vi "INIT.vi"(8 "error in (no error)":errorcluster, 11 "UV-VIS_AVANTES in":refnum<class "UV-VIS_AVANTES.lvclass">) -> (0 "error out":errorcluster, 3 "UV-VIS_AVANTES out":refnum<class "UV-VIS_AVANTES.lvclass">)   [LabVIEW 2020, in "UV-VIS_AVANTES.lvclass"]
uses:
  UV-VIS_AVANTES.lvclass
  C:/dev/TRANCON/Classes/GeneralFunctionality/GeneralFunctionality.lvclass
  C:/dev/TRANCON/Classes/Detector/Detector.lvclass
  GeneralFunctionality/GeneralFunctionality.lvclass/GeneralFunctionality.ctl
  UV-VIS_AVANTES.lvclass/UV-VIS_AVANTES.ctl
  Detector.lvclass/Detector.ctl
  dependecies/globalVarII.vi
  Config/Config.lvclass
  Detector.lvclass
  GeneralFunctionality/GeneralFunctionality.lvclass
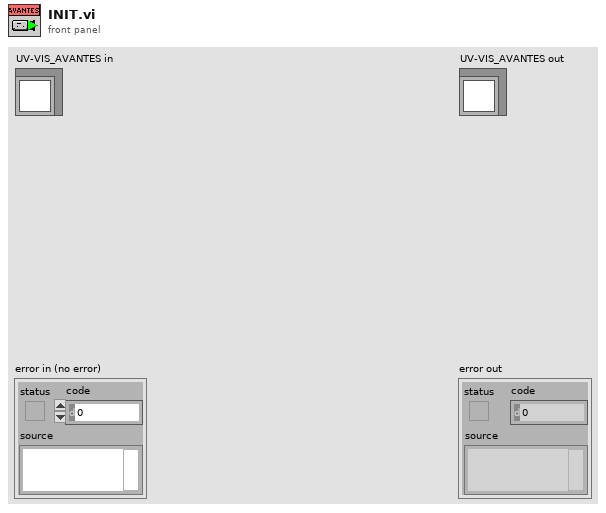
[diagram p1: front panel]
types:
  T1 = typedef "UV-VIS_AVANTES.lvclass/def_parameters.ctl" = cluster{"Len":u16, "ConfigVersion":u16, "UserFriendlyId":u8[], "DetectorType":cluster{"SensorType":u8, "NrPixels":u16, "Fit":sgl[], "NLEnable":u8, "NLCorrect":dbl[], "LowNLCounts":dbl, "HighNLCounts":dbl, "Gain":sgl[], "Reserved":sgl, "Offset":sgl[], "Extern Offset":sgl, "DefectivePixels":u16[]}, "IrradianceType":cluster{"SpectrumCalibrationType":cluster{"SmoothingType":cluster{"m_SmoothPix":u16, "SmoothModel":u8}, "CalInttime":sgl, "CalibConvers":sgl[]}, "CalibrationType":u8, "FiberDiameter":i32}, "SpectrumCalibrationType":cluster{"SmoothingType":cluster{"m_SmoothPix":u16, "SmoothModel":u8}, "CalInttime":sgl, "CalibConvers":sgl[]}, "SpectrumCorrectionType":sgl[], "StandAloneType":cluster{"StandAloneType":u8, "MeasConfigType":cluster{"StartPixel":u16, "StopPixel":u16, "IntegrationTime":sgl, "IntegrationDelay":u32, "NrAverages":u32, "DarkCorrectionType":cluster{"Enable CorDynDark":u8, "ForgetPercentage":u8}, "SmoothingType":cluster{"SmoothPix":u16, "SmoothModel":u8}, "SatDetection":u8, "TriggerType":cluster{"Trigger Mode":u8, "Trigger Source":u8, "Trigger SourceType":u8}, "ControlSettingsType":cluster{"StrobeControl":u16, "LaserDelay":u32, "LaserWidth":u32, "LaserWaveLength":sgl, "StoreToRam":u16}}, "Nmsr":i16}, "DynamicStorageType":cluster{"Nmsr":i32, "Reserved":u8[]}, "TempSensorType":sgl[], "TecControlType":cluster{"Enable":u8, "Setpoint":sgl, "Fit[NR_DAC_POL_COEF]":sgl[]}, "ProcessControlType":cluster{"AnalogLow":sgl[], "AnalogHigh":sgl[], "DigitalLow":sgl[], "DigitalHigh":sgl[]}, "EthernetSettingsType":cluster{"IpAddr":u32, "NetMask":u32, "Gateway":u32, "DhcpEnabled":u8, "TcpPort":u16, "LinkStatus":u8}, "Reserved":u8[]}
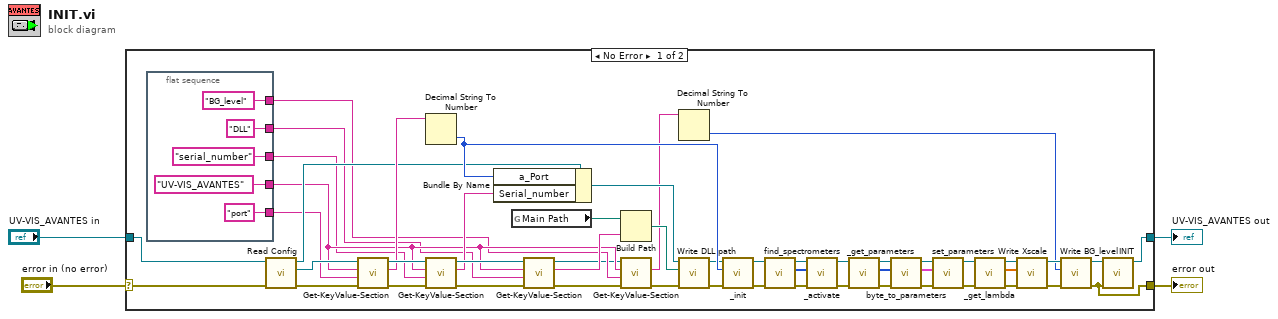
[diagram p0: block diagram]
diagram:
  n1 = case shown="No Error" "error in (no error)" {
    selector: "error in (no error)" -> [w44 w61]
    tunnel: [w32 w62] -> w3
    tunnel: "UV-VIS_AVANTES in" -> [w50 w62]
    tunnel: [w5 w61] -> w1
    frame No Error {
      n2 = flat-sequence {
        tunnel: ["UV-VIS_AVANTES" ("Section")] -> w11
        tunnel: ["serial_number" ("Key")] -> w10
        tunnel: ["BG_level" ("Key")] -> w9
        tunnel: ["port" ("Key")] -> w8
        tunnel: ["DLL" ("Key")] -> w7
        frame #0 {
        }
      }
      n3 = call "Read Config.vi"("error in (no error)"=w44, "GeneralFunctionality en entrée"=w50) -> ("error out"=w49:errorcluster, "Config.lvclass"=w51:refnum<class "Config.lvclass">, "GeneralFunctionality en sortie"=w43:refnum<class "UV-VIS_AVANTES.lvclass">)  [unwired: 7 in]
      n4 = call-dynamic "Get-KeyValue-Section.vi"("error in (no error)"=w49, "Key"=w8, "Section"=w11, "Config in"=w51) -> ("error out"=w48:errorcluster, "Value"=w46:string, "Config out"=w47:refnum<class "Config.lvclass">)  [unwired: 5 in]
      n5 = Decimal String To Number(string=w46) -> (number=w45:i32)  [unwired: 2 in, 1 out]
      n6 = call-dynamic "Get-KeyValue-Section.vi"("error in (no error)"=w48, "Key"=w10, "Section"=w11, "Config in"=w47) -> ("error out"=w28:errorcluster, "Value"=w19:string, "Config out"=w27:refnum<class "Config.lvclass">)  [unwired: 5 in]
      n7 = Bundle By Name(cluster=w43, "a_Port"=w45, "Serial_number"=w19) -> (w31:refnum<class "UV-VIS_AVANTES.lvclass">)
      n8 = global read "globalVarII.vi" "Main Path"() -> (w20:path)
      n9 = call-dynamic "Get-KeyValue-Section.vi"("error in (no error)"=w28, "Key"=w7, "Section"=w11, "Config in"=w27) -> ("error out"=w15:errorcluster, "Value"=w26:string, "Config out"=w6:refnum<class "Config.lvclass">)  [unwired: 5 in]
      n10 = Build Path(base path=w20, name or relative path=w26) -> (appended path=w25:path)
      n11 = call-dynamic "Get-KeyValue-Section.vi"("error in (no error)"=w15, "Key"=w9, "Section"=w11, "Config in"=w6) -> ("error out"=w14:errorcluster, "Value"=w13:string)  [unwired: 5 in, 1 out]
      n12 = Decimal String To Number(string=w13) -> (number=w12:i32)  [unwired: 2 in, 1 out]
      n13 = call "Write DLL path.vi"("error in (no error)"=w14, "DLL path"=w25, "Detector in"=w31) -> ("error out"=w29:errorcluster, "Detector out"=w30:refnum<class "UV-VIS_AVANTES.lvclass">)  [unwired: 7 in]
      n14 = call "_init.vi"("error in (no error)"=w29, "a_Port"=w45, "UV-VIS_AVANTES in"=w30) -> ("error out"=w53:errorcluster, "UV-VIS_AVANTES out"=w54:refnum<class "UV-VIS_AVANTES.lvclass">)  [unwired: 6 in, 1 out]
      n15 = call "find_spectrometers.vi"("error in (no error)"=w53, "UV-VIS_AVANTES in"=w54) -> ("error out"=w52:errorcluster, "List Output"=w42:u8[], "UV-VIS_AVANTES out"=w55:refnum<class "UV-VIS_AVANTES.lvclass">)  [unwired: 7 in]
      n16 = call "_activate.vi"("error in (no error)"=w52, "a_pDeviceId IN"=w42, "UV-VIS_AVANTES in"=w55) -> ("error out"=w36:errorcluster, "UV-VIS_AVANTES out"=w37:refnum<class "UV-VIS_AVANTES.lvclass">)  [unwired: 7 in]
      n17 = call "_get_parameters.vi"("error in (no error)"=w36, "UV-VIS_AVANTES in"=w37) -> ("error out"=w41:errorcluster, "DeviceParam"=w21:u8[], "UV-VIS_AVANTES out"=w38:refnum<class "UV-VIS_AVANTES.lvclass">)  [unwired: 7 in]
      n18 = call "byte_to_parameters.vi"("error in (no error)"=w41, "DeviceParam"=w21, "UV-VIS_AVANTES in"=w38) -> ("error out"=w39:errorcluster, "parameters cluster"=w24:T1, "UV-VIS_AVANTES out"=w40:refnum<class "UV-VIS_AVANTES.lvclass">)  [unwired: 6 in]
      n19 = call "set_parameters.vi"("error in (no error)"=w39, "AVS_parameters"=w24, "UV-VIS_AVANTES in"=w40) -> ("error out"=w22:errorcluster, "UV-VIS_AVANTES out"=w23:refnum<class "UV-VIS_AVANTES.lvclass">)  [unwired: 7 in]
      n20 = call "_get_lambda.vi"("error in (no error)"=w22, "UV-VIS_AVANTES in"=w23) -> ("error out"=w33:errorcluster, "a_pWaveLength"=w35:dbl[], "UV-VIS_AVANTES out"=w34:refnum<class "UV-VIS_AVANTES.lvclass">)  [unwired: 7 in]
      n21 = call "Write Xscale.vi"("error in (no error)"=w33, "Xscale"=w35, "Detector en entrée"=w34) -> ("error out"=w16:errorcluster, "Detector en sortie"=w18:refnum<class "UV-VIS_AVANTES.lvclass">)  [unwired: 7 in]
      n22 = call-dynamic "Write BG_level.vi"("error in (no error)"=w16, "BG_level"=w12, "Detector in"=w18) -> ("error out"=w5:errorcluster, "Detector out"=w17:refnum<class "UV-VIS_AVANTES.lvclass">)  [unwired: 7 in]
      n23 = call-parent "INIT.vi"("error in (no error)"=w5, "Detector in"=w17) -> ("Detector out"=w32:refnum<class "UV-VIS_AVANTES.lvclass">)  [unwired: 8 in, 1 out]
    }
    frame Error {
    }
  }
  "error out" <- w1
  "UV-VIS_AVANTES out" <- w3
